vi "_CSMOFGV Get.vi"(8 "Error In":errorcluster caption="error in (no error)", 10 "Message":string, 11 "Name (\"\" to Use UUID) In":string) -> (0 "error out":errorcluster, 3 "CSM-Obj":T1={"info"={"Module Name"="", "Requested Name"="", "Group Name"="", "Mode"=enum."Stand Alone", "Allowed Messages"=[]}, "Refs"={"WatchDogQ"=refnum, "CSMDataDVR"=refnum, "Queue"={"HPriorityQ"=refnum, "LowPriorityQ"=refnum}, "GroupDataDVR"=refnum, "TagMap"=refnum, "ExitEvent"=refnum, "NewStateEvent"=refnum, "StatusEvent"=refnum, "InterruptEvent"=refnum}}, 4 "Name":string)   [LabVIEW 2017, in "Communicable State Machine.lvlib"]
uses:
  Communicable State Machine.lvlib
  _CSMObj.ctl
  _CSMObj-Info.ctl
  Typedef/_CSM_MODE.ctl
  _CSMObj-Refs.ctl
  _CSMObj-Data.ctl
  Typedef/_CSM_MSG_TYPE.ctl
  Priority Queue/Priority Queue.ctl
  Typedef/_Cross CSM State Data.ctl
  Typedef/_Cross CSM State Response.ctl
  Typedef/_CSM_Response Source Message.ctl
  Priority Queue/def-Data(LowPRI-Q).ctl
  _CSMObj-ModeData.ctl
  Typedef/_CSM Status Change Event Data.ctl
  _CSMOFGVOPER.ctl
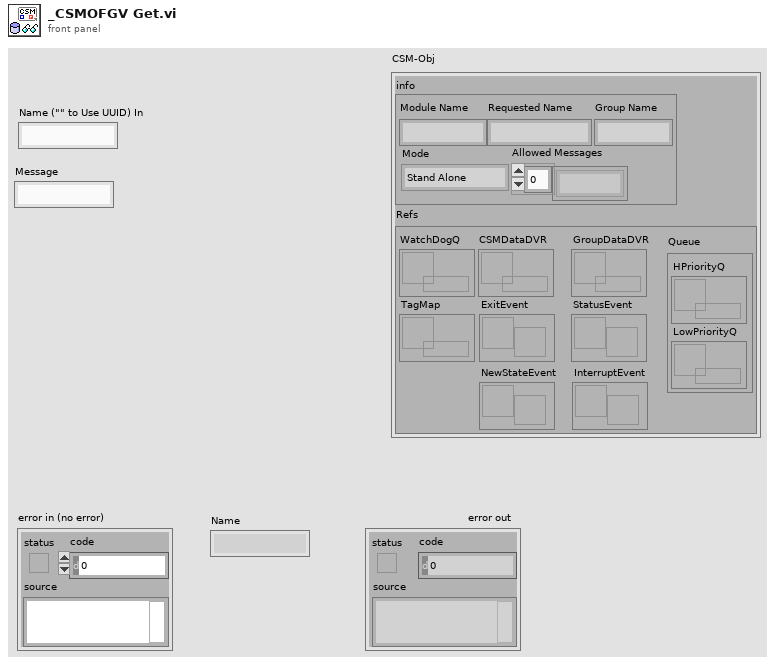
[diagram p1: front panel]
types:
  T1 = typedef "Communicable State Machine.lvlib/_CSMObj.ctl" = cluster{"info":T2, "Refs":T4}
  T2 = typedef "Communicable State Machine.lvlib/_CSMObj-Info.ctl" = cluster{"Module Name":string, "Requested Name":string, "Group Name":string, "Mode":T3, "Allowed Messages":string[]}
  T3 = typedef "Communicable State Machine.lvlib/_CSM_MODE.ctl" = enum16{"Not Exist", "Stand Alone", "CSM", "Worker", "Worker Agent", "Chain Node", "Chain"}
  T4 = typedef "Communicable State Machine.lvlib/_CSMObj-Refs.ctl" = cluster{"WatchDogQ":refnum<queue>, "CSMDataDVR":refnum<data-value>, "Queue":T5, "GroupDataDVR":refnum<data-value>, "TagMap":refnum<data-value>, "ExitEvent":refnum<user-event>, "NewStateEvent":refnum<user-event>, "StatusEvent":refnum<user-event>, "InterruptEvent":refnum<user-event>}
  T5 = typedef "Communicable State Machine.lvlib/Priority Queue.ctl" = cluster{"HPriorityQ":refnum<queue>, "LowPriorityQ":refnum<queue>}
  T6 = typedef "Communicable State Machine.lvlib/_CSMOFGVOPER.ctl" = enum16{"Create If not Exist", "Get By Name", "List", "Check If Name Exists", "Release", "Module Status", "Create Status Event Handler", "Destroy Status Event Handler", "Clear Invalid Objs"}
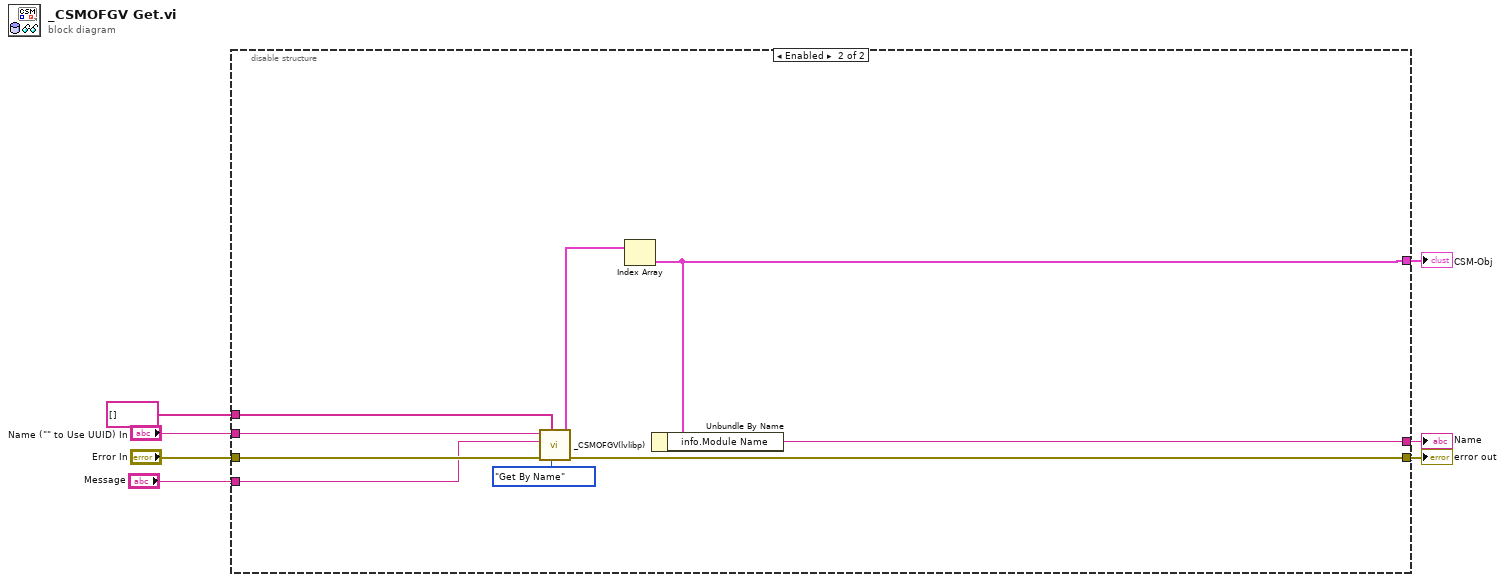
[diagram p0: block diagram]
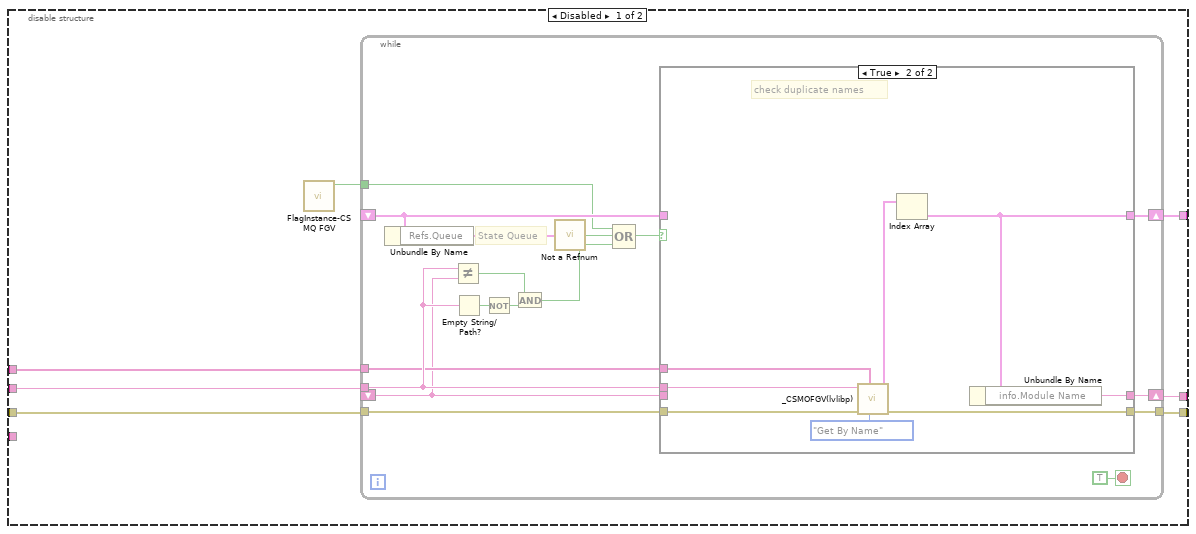
[diagram p2: hidden frame]
diagram:
  n1 = disable-structure shown="Enabled" {
    disable-tunnel: [w14 w45] -> w7
    disable-tunnel: "Error In" -> [w13 w47]
    disable-tunnel: [w12 w46] -> w5
    disable-tunnel: "Name (\"\" to Use UUID) In" -> [w11 w49]
    disable-tunnel: [w10 w44] -> w3
    disable-tunnel: string[] [] ("Allowed Messages(Empty for all)") -> [w9 w48]
    disable-tunnel: "Message" -> [_ w43]
    frame Disabled {
      n2 = call "FlagInstance-CSMQ FGV.vi"() -> ("Changed"=w8:bool)  [unwired: 10 in, 1 out]
      n3 = while {
        shift-right: [w29] -> w14
        shift-left: _ -> [w15]
        shift-right: [w28] -> w10
        shift-left: _ -> [w22]
        tunnel: w13 -> [w27]
        tunnel: [w26] -> w12
        tunnel: w11 -> [w23]
        tunnel: w8 -> [w17]
        tunnel: w9 -> [w16]
        stop <- TRUE stop-if-true
        # "State Queue"
        n4 = Unbundle By Name(w22) -> ("Refs.Queue"=w21:T5)
        n5 = Not Equal?(x=w23, y=w15) -> (x != y?=w20:bool)
        n6 = Empty String/Path?(string/path=w23) -> (empty?=w19:bool)
        n7 = Not(x=w19) -> (.not. x?=w18:bool)
        n8 = And(x=w20, y=w18) -> (x .and. y?=w24:bool)
        n9 = call "Not a Refnum.vi"("Priority Queue.lvclass"=w21) -> ("NaN/Path/Refnum?"=w30:bool)  [unwired: 4 in]
        n10 = Compound Arithmetic op=OR(w17, w30, w24) -> (w25:bool)
        n11 = case shown="True" w25 {
          tunnel: w15 -> [w34 _]
          tunnel: [w34 w35] -> w29
          tunnel: [w33 w36] -> w28
          tunnel: w22 -> [w33 _]
          tunnel: w27 -> [w32 w38]
          tunnel: [w32 w40] -> w26
          tunnel: w23 -> [_ w39]
          tunnel: w16 -> [_ w37]
          frame False {
          }
          frame True {
            # "check duplicate names"
            n12 = call "_CSMOFGV(lvlibp).vi"("Operation"=_CSMOFGVOPER."Get By Name", "Allowed Messages (Empty For All)"=w37, "Error In"=w38, "Name (\"\" to Use UUID) In"=w39) -> ("error out"=w40:errorcluster, "Array"=w42:T1[])  [unwired: 5 in, 1 out]
            n13 = Index Array(array=w42) -> (element=w36:T1)  [unwired: 1 in]
            n14 = Unbundle By Name(w36) -> ("info.Module Name"=w35:string)
          }
        }
      }
    }
    frame Enabled {
      n15 = call "_CSMOFGV(lvlibp).vi"("Operation"=_CSMOFGVOPER."Get By Name", "Allowed Messages (Empty For All)"=w48, "Error In"=w47, "Reference"=w43, "Name (\"\" to Use UUID) In"=w49) -> ("error out"=w46:errorcluster, "Array"=w51:T1[])  [unwired: 4 in, 1 out]
      n16 = Index Array(array=w51) -> (element=w44:T1)  [unwired: 1 in]
      n17 = Unbundle By Name(w44) -> ("info.Module Name"=w45:string)
    }
  }
  "error out" <- w5
  "CSM-Obj" <- w3
  "Name" <- w7
